vi "Controls.vi"() -> ()   [LabVIEW 2017]
panel:
  out "DI2.31":bool
  out "DI2.30":bool
  out "DI2.29":bool
  out "DI2.28":bool
  out "DI2.27":bool
  out "DI2.26":bool
  out "DI2.25":bool
  out "DI2.24":bool
  out "DI2.23":bool
  out "RS_Rejection_4_Rear":bool
  out "RS_Rejection_3_Rear":bool
  out "RS_Rejection_2_Rear":bool
  out "RS_Rejection_1_Rear":bool
  out "RS_Clamping_CYL":bool
  out "RS_Measurement_4_Rear":bool
  out "RS_Measurement_3_Rear":bool
  out "RS_Measurement_2_Rear":bool
  out "RS_Measurement_1_Rear":bool
  out "RS_Clamping _Rear":bool
  out "RS_Cutting_Rear":bool
  out "RS_Insertion_Clamping_CYL":bool
  out "RS_Insertion _4_Front":bool
  out "RS_Insertion _4_Rear":bool
  out "RS_Insertion _3_Front":bool
  out "RS_Insertion _3_Rear":bool
  out "RS_Insertion _2_Front":bool
  out "RS_Insertion _2_Rear":bool
  out "RS_Insertion_1_Front":bool
  out "RS_Insertion_1_Rear":bool
  out "RS_Gating CYL_Rear":bool
  out "RS_Agitatator_2_Rear":bool
  out "RS_Agitatator_1_Rear":bool
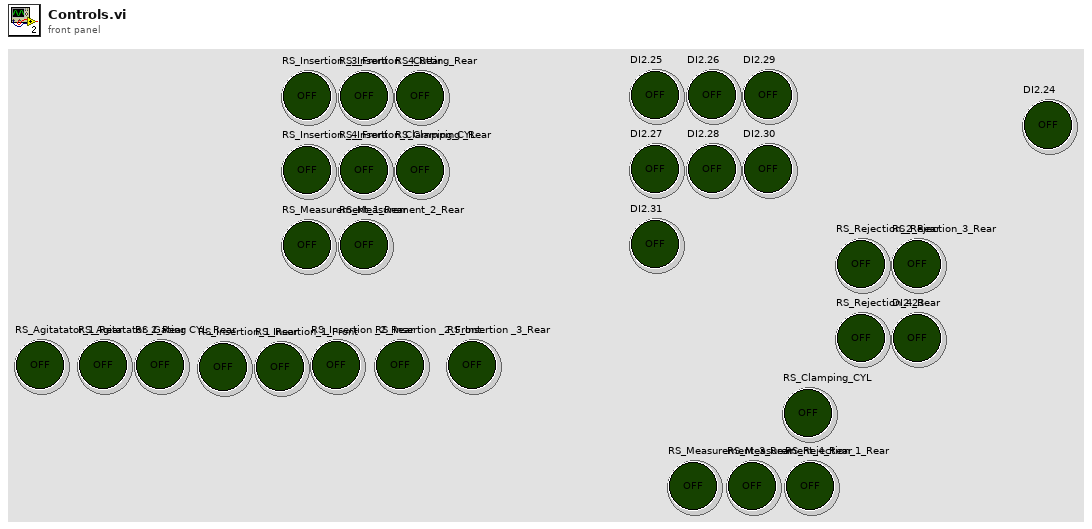
[diagram p1: front panel]
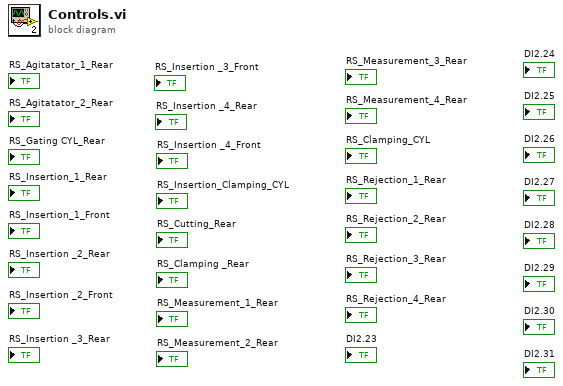
[diagram p0: block diagram]
diagram:
